vi "Industrial Turbine Model.vi"(0 "Turbine Build Specifications":T1={"Length (m)"=5, "Width (m)"=5, "Height (m)"=5, "Condenser Layers"=1, "Rotor Height"=1, "Vents"=5, "Condensers"=5} {"Condensers" min=0 max=218 step=1; "Vents" min=-75 max=345 step=1; "Rotor Height" min=0 max=14 step=1; "Condenser Layers" min=0 max=14 step=1; "Height (m)" min=4 max=18 step=1; "Width (m)" min=5 max=17 step=2; "Length (m)" min=5 max=17 step=2}) -> (10 "Energy Production (FE/t)":ext format="%.2f", 11 "Turbine Build Properties":T2 {"Energy Capacity (FE)" format="%.2f"}, 13 "Energy Production\nEfficiency (η)":ext, 14 "Flow (mB/t)":i64, 15 "Water Return (mB/t)":i64, 16 "Vents Limiting":bool, 17 "Dispersers Limiting":bool, 18 "Blades Limiting":bool, 19 "Coils Limiting":bool)   [LabVIEW 2026]
uses:
  Turbine Build Properties.ctl
  Turbine Build Specifications.ctl
  bbb8b91a-5175-7941-9f9e-431f1dc08699.vi
panel:
  out "Max Condenser Layers":i32
  out "Max Vents":i32 max=8
  out "Return Limited":bool
  out "Max Condensers":i32 max=8
  out "Maximum Height (m)":i32
  out "Maximum Rotor Height (m)":i32
  # "Industrial Turbine Build"
  # "Industrial Turbine Properties"
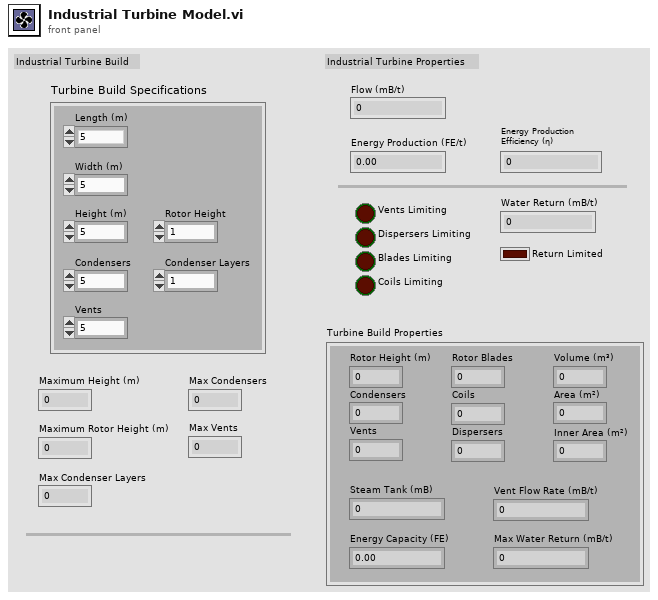
[diagram p1: front panel]
types:
  T1 = typedef "Turbine Build Specifications.ctl" = cluster{"Length (m)":i32, "Width (m)":i32, "Height (m)":i32, "Condenser Layers":i32, "Rotor Height":i32, "Vents":i32, "Condensers":i32}
  T2 = typedef "Turbine Build Properties.ctl" = cluster{"Volume (m³)":i32, "Rotor Height (m)":i32, "Condensers":i32, "Vents":i32, "Rotor Blades":i32, "Coils":i32, "Dispersers":i32, "Steam Tank (mB)":i64, "Energy Capacity (FE)":ext, "Vent Flow Rate (mB/t)":dbl, "Max Water Return (mB/t)":i32, "Area (m²)":i32, "Inner Area (m²)":i32}
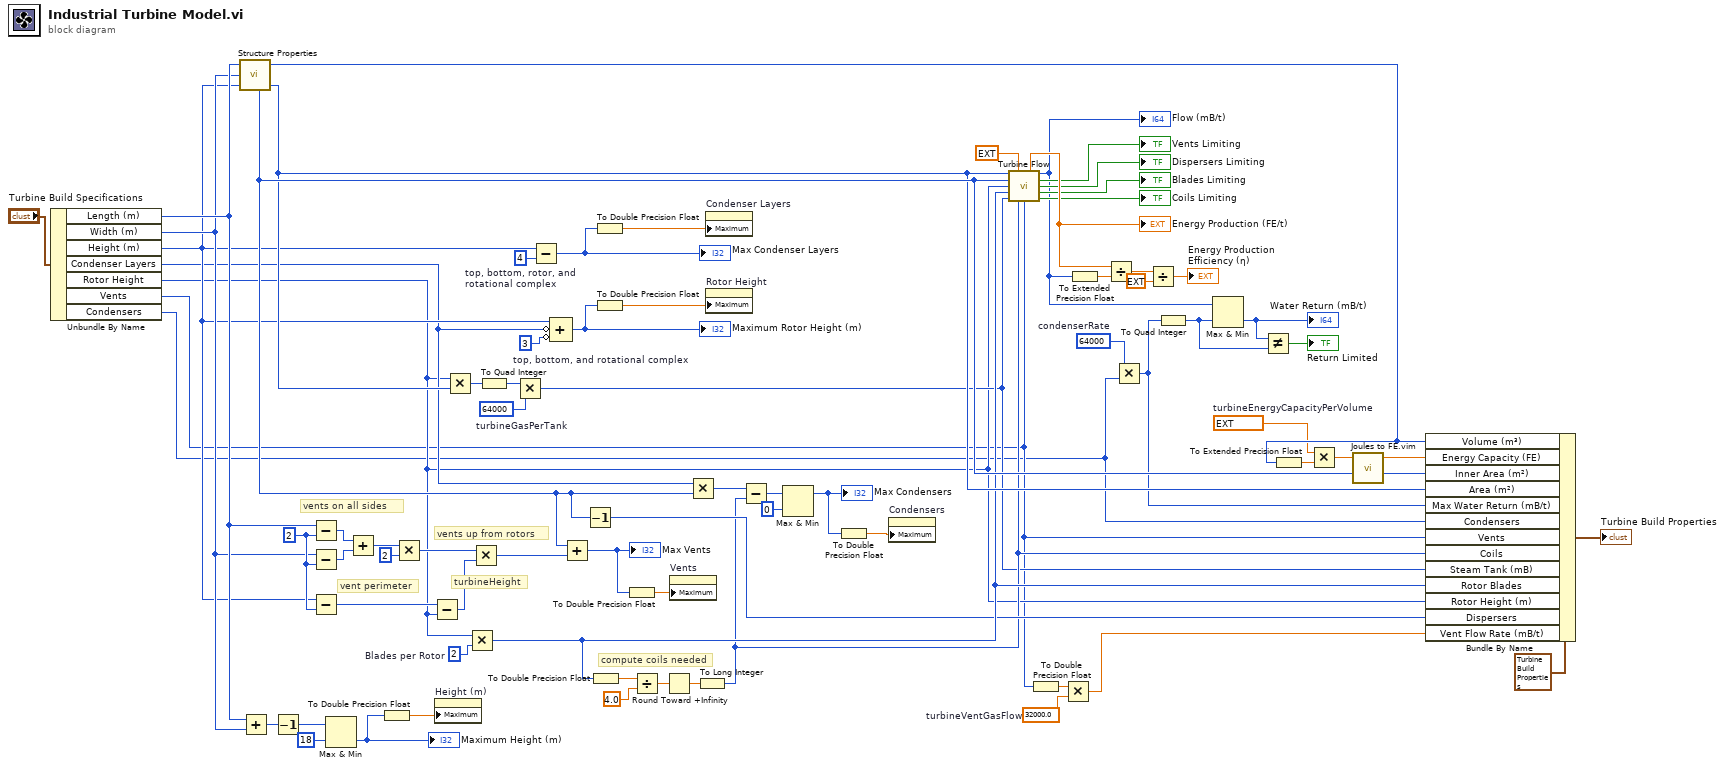
[diagram p0: block diagram]
diagram:
  w28 = 2 ("y")
  w34 = 4  # top, bottom, rotor, and rotational complex
  w10 = ext 16000000.0  # turbineEnergyCapacityPerVolume
  w36 = 3  # top, bottom, and rotational complex
  w56 = 64000  # condenserRate
  w61 = 32000.0  # turbineVentGasFlow
  w62 = 2  # Blades per Rotor
  w66 = i64 64000  # turbineGasPerTank
  # "compute coils needed"
  # "turbineHeight"
  # "vent perimeter"
  # "vents up from rotors"
  # "vents on all sides"
  n1 = Unbundle By Name("Turbine Build Specifications") -> ("Length (m)"=w7:i32, "Width (m)"=w6:i32, "Height (m)"=w5:i32, "Condenser Layers"=w4:i32, "Rotor Height"=w3:i32, "Vents"=w2:i32, "Condensers"=w1:i32)
  n2 = call "Structure Properties.vi"("Length"=w7, "Width"=w6, "Height"=w5) -> ("Volume"=w12:i32, "Inner Area"=w74:i32, "Area"=w73:i32)  [unwired: 2 in, 2 out]
  n3 = Add(x=w7, y=w6) -> (x+y=w38:i32)
  n4 = Decrement(x=w38) -> (x-1=w68:i32)
  n5 = Subtract(x=w7, y=w28) -> (x-y=w27:i32)
  n6 = Subtract(x=w6, y=w28) -> (x-y=w26:i32)
  n7 = Subtract(x=w5, y=w28) -> (x-y=w46:i32)
  n8 = Max & Min(x=w68, y=18) -> (min(x,y)=w65:i32)  [unwired: 1 out]
  "Maximum Height (m)" <- w65
  n9 = Add(x=w27, y=w26) -> (x+y=w25:i32)
  n10 = To Double Precision Float(number=w65) -> (double precision float=w64:dbl)
  n11 = Multiply(x=w25, y=2) -> (x*y=w23:i32)
  n12 = Subtract(x=w46, y=w3) -> (x-y=w48:i32)
  n13 = property on="Height (m)" class="DigNum (strict)"("Maximum"=w64) -> ()  [unwired: 2 in, 2 out]
  n14 = Multiply(x=w3, y=w73) -> (x*y=w67:i32)
  n15 = Multiply(x=w3, y=w62) -> (x*y=w72:i32)
  n16 = Multiply(x=w23, y=w48) -> (x*y=w22:i32)
  n17 = To Quad Integer(1:w67) -> (0:w30:i64)
  n18 = Multiply(x=w30, y=w66) -> (x*y=w13:i64)
  n19 = Subtract(x=w5, y=w34) -> (x-y=w35:i32)
  "Max Condenser Layers" <- w35
  n20 = Compound Arithmetic op=ADD(w5, invert w4, invert w36) -> (w37:i32)
  "Maximum Rotor Height (m)" <- w37
  n21 = Add(x=w74, y=w22) -> (x+y=w18:i32)
  "Max Vents" <- w18
  n22 = Decrement(x=w74) -> (x-1=w71:i32)
  n23 = To Double Precision Float(number=w72) -> (double precision float=w60:dbl)
  n24 = To Double Precision Float(number=w35) -> (double precision float=w33:dbl)
  n25 = To Double Precision Float(number=w37) -> (double precision float=w63:dbl)
  n26 = To Double Precision Float(number=w18) -> (double precision float=w47:dbl)
  n27 = Divide(x=w60, y=4.0) -> (x/y=w58:dbl)
  n28 = Round Toward +Infinity(x=w58) -> (ceil(x): smallest int >= x=w57:dbl)
  n29 = property on="Vents" class="DigNum (strict)"("Maximum"=w47) -> ()  [unwired: 2 in, 2 out]
  n30 = Multiply(x=w4, y=w74) -> (x*y=w29:i32)
  n31 = To Long Integer(number=w57) -> (32bit integer=w70:i32)
  n32 = property on="Condenser Layers" class="DigNum (strict)"("Maximum"=w33) -> ()  [unwired: 2 in, 2 out]
  n33 = property on="Rotor Height" class="DigNum (strict)"("Maximum"=w63) -> ()  [unwired: 2 in, 2 out]
  n34 = Subtract(x=w29, y=w70) -> (x-y=w20:i32)
  n35 = Max & Min(x=w20, y=0) -> (max(x,y)=w19:i32)  [unwired: 1 out]
  "Max Condensers" <- w19
  n36 = To Double Precision Float(number=w19) -> (double precision float=w55:dbl)
  n37 = property on="Condensers" class="DigNum (strict)"("Maximum"=w55) -> ()  [unwired: 2 in, 2 out]
  n38 = call "Turbine Flow.vi"("Structure Area (m²)"=w73, "Energy Needed (FE)"=ext inf, "Inner Area (m²)"=w74, "Rotor Height (m)"=w3, "Blades"=w72, "Stored Gas (mB/t)"=w13, "Coils"=w70, "Vents"=w2) -> ("Energy Production (FE/t)"=w75:ext, "Flow (mB/t)"=w45:i64, "Vents Limiting"=→"Vents Limiting":bool, "Dispersers Limiting"=→"Dispersers Limiting":bool, "Blades Limiting"=→"Blades Limiting":bool, "Coils Limiting"=→"Coils Limiting":bool)  [unwired: 1 in, 1 out]
  "Energy Production (FE/t)" <- w75
  "Flow (mB/t)" <- w45
  n39 = To Double Precision Float(number=w2) -> (double precision float=w31:dbl)
  n40 = Multiply(x=w31, y=w61) -> (x*y=w14:dbl)
  n41 = To Extended Precision Float(1:w45) -> (0:w44:ext)
  n42 = Divide(x=w75, y=w44) -> (x/y=w43:ext)
  n43 = Multiply(x=w56, y=w1) -> (x*y=w15:i32)
  n44 = Divide(x=w43, y=ext 4.0) -> (x/y=→"Energy Production\nEfficiency (η)":ext)
  n45 = To Quad Integer(1:w15) -> (0:w32:i64)
  n46 = Max & Min(x=w45, y=w32) -> (min(x,y)=w50:i64)  [unwired: 1 out]
  "Water Return (mB/t)" <- w50
  n47 = Not Equal?(x=w50, y=w32) -> (x != y?=→"Return Limited":bool)
  n48 = To Extended Precision Float(1:w12) -> (0:w39:ext)
  n49 = Multiply(x=w10, y=w39) -> (x*y=w40:ext)
  n50 = call "Joules to FE.vim"("J"=w40) -> ("FE"=w11:ext)  [unwired: 4 in]
  n51 = Bundle By Name(cluster=T2 {"Volume (m³)"=0, "Rotor Height (m)"=0, "Condensers"=0, "Vents"=0, "Rotor Blades"=0, "Coils"=0, "Dispersers"=0, "Steam Tank (mB)"=0, "Energy Capacity (FE)"=0.0, "Vent Flow Rate (mB/t)"=0.0, "Max Water Return (mB/t)"=0, "Area (m²)"=0, "Inner Area (m²)"=0} ("Turbine Build Properties"), "Volume (m³)"=w12, "Energy Capacity (FE)"=w11, "Inner Area (m²)"=w74, "Area (m²)"=w73, "Max Water Return (mB/t)"=w15, "Condensers"=w1, "Vents"=w2, "Coils"=w70, "Steam Tank (mB)"=w13, "Rotor Blades"=w72, "Rotor Height (m)"=w3, "Dispersers"=w71, "Vent Flow Rate (mB/t)"=w14) -> (→"Turbine Build Properties":T2)
